vi "gcode_v2.vi"() -> ()   [LabVIEW 2020]
uses:
  bee2abb7-c490-4ad6-bfc0-30ed72578e14.vi
panel:
  in  "Convert":bool
  in  "Load":bool
  in  "File Path":path
  in  "Gcode":string
  out "Paths":cluster{"x":dbl, "y":dbl}[](array[cluster])
  out "Preview":cluster{dbl[], dbl[]}[](graph)
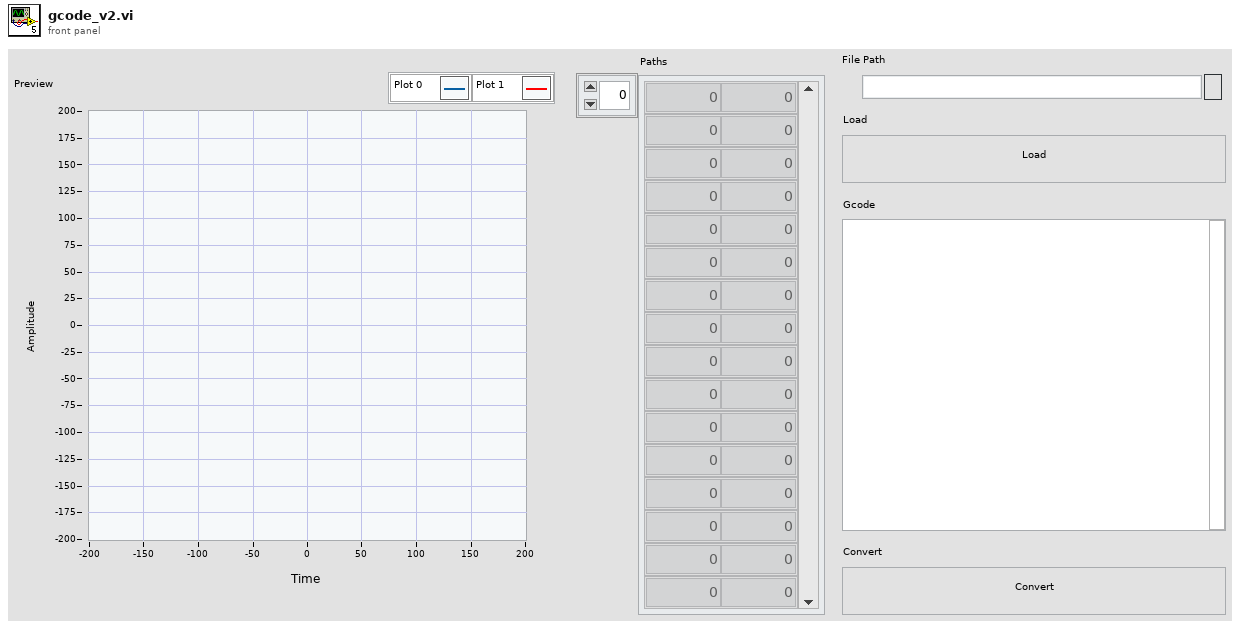
[diagram p1: front panel]
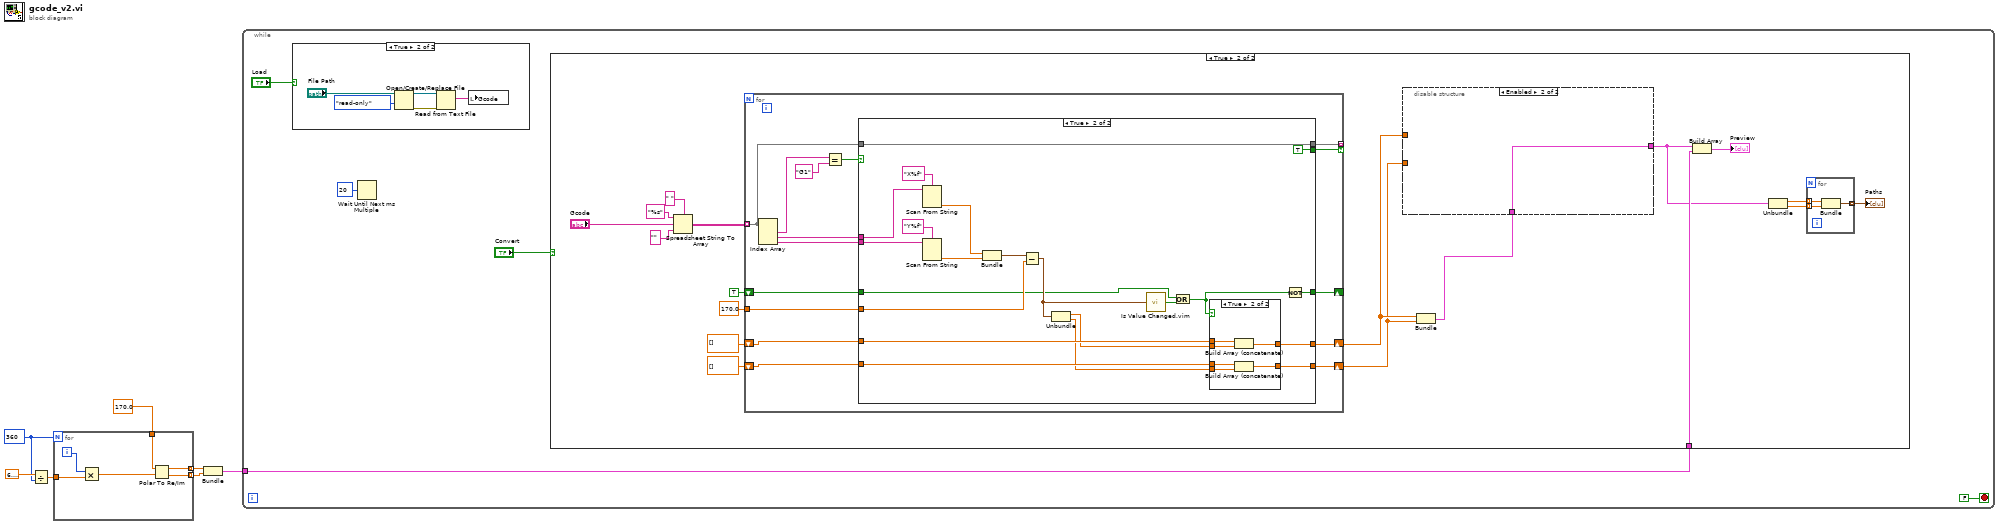
[diagram p0: block diagram]
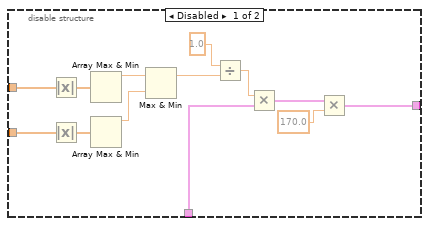
[diagram p5: hidden frame]
diagram:
  w6 = 360
  n1 = Divide(x=6.283185307179586, y=w6) -> (x/y=w5:dbl)
  n2 = for {
    N: w6 -> [_]
    tunnel: [w13] -> w3 mode=indexing
    tunnel: [w12] -> w2 mode=indexing
    tunnel: w5 -> [w10]
    tunnel: 170.0 ("r") -> [w8]
    i -> [w11]
    n3 = Multiply(x=w11, y=w10) -> (x*y=w9:dbl)
    n4 = Polar To Re/Im(2:w9, 3:w8) -> (0:w12:dbl, 1:w13:dbl)
  }
  n5 = Bundle(w3, w2) -> (w1:cluster{dbl[], dbl[]})  [unwired: 1 in]
  n6 = while {
    tunnel: w1 -> [w17]
    stop <- FALSE stop-if-true
    n7 = case shown="True" "Load" {
      frame False {
      }
      frame True {
        n8 = Open/Create/Replace File(file path (use dialog)="File Path", access (0:read/write)=enum16{"read/write", "read-only", "write-only"}."read-only") -> (refnum out=w102:refnum<file>, error out=w103:errorcluster)  [unwired: 4 in, 1 out]
        n9 = Read from Text File(file (use dialog)=w102, error in=w103) -> (text=w101:string)  [unwired: 2 in, 3 out]
        n10 = local write "Gcode"(w101) -> ()
      }
    }
    n11 = Wait Until Next ms Multiple(millisecond multiple=u32 20) -> ()  [unwired: 1 out]
    n12 = case shown="True" "Convert" {
      tunnel: w17 -> [_ w21]
      frame False {
      }
      frame True {
        n13 = Spreadsheet String To Array(delimiter (Tab)=" ", format string="%s", spreadsheet string="Gcode", array type (2D Dbl)="" ("delimiter (Tab)")) -> (array=w28:string[][])
        n14 = for {
          shift-right: [w49] -> w26
          shift-left: dbl[] [] -> [w51]
          shift-right: [w48] -> w25
          shift-left: dbl[] [] -> [w50]
          tunnel: w28 -> [w40] mode=indexing
          tunnel: 170.0 -> [w45]
          tunnel: [w41] -> _ mode=indexing if=w39
          shift-right: [w38] -> _
          shift-left: TRUE -> [w37]
          n15 = Index Array(array=w40) -> (element #1=w44:string, element #2=w47:string, element #3=w46:string)  [unwired: 3 in]
          n16 = Equal?(x=w44, y="G1") -> (x = y?=w42:bool)
          n17 = case shown="True" w42 {
            tunnel: w51 -> [w54 w75]
            tunnel: w50 -> [w53 w74]
            tunnel: [w54 w73] -> w49
            tunnel: [w53 w72] -> w48
            tunnel: w47 -> [_ w68]
            tunnel: w46 -> [_ w67]
            tunnel: w45 -> [_ w64]
            tunnel: [_ w60] -> w41
            tunnel: w40 -> [_ w60]
            tunnel: [_ TRUE] -> w39
            tunnel: [w52 w55] -> w38
            tunnel: w37 -> [w52 w57]
            frame False {
            }
            frame True {
              n18 = Scan From String(format string="X%f", input string=w68) -> (output 1=w70:dbl)  [unwired: 3 in, 3 out]
              n19 = Scan From String(format string="Y%f", input string=w67) -> (output 1=w66:dbl)  [unwired: 3 in, 3 out]
              n20 = Bundle(w70, w66) -> (w65:cluster{dbl, dbl})  [unwired: 1 in]
              n21 = Subtract(x=w65, y=w64) -> (x-y=w63:cluster{dbl, dbl})
              n22 = Unbundle(w63) -> (w62:dbl, w61:dbl)
              n23 = call "Is Value Changed.vim"("value"=w63) -> ("changed or first call?"=w58:bool)
              n24 = Or(x=w57, y=w58) -> (x .or. y?=w56:bool)
              n25 = case shown="True" w56 {
                tunnel: w62 -> [_ w83]
                tunnel: w61 -> [_ w82]
                tunnel: [w77 w81] -> w73
                tunnel: [w76 w80] -> w72
                tunnel: w75 -> [w77 w79]
                tunnel: w74 -> [w76 w78]
                frame False {
                }
                frame True {
                  n26 = Build Array (concatenate)(w79, w83) -> (w81:dbl[])
                  n27 = Build Array (concatenate)(w78, w82) -> (w80:dbl[])
                }
              }
              n28 = Not(x=w56) -> (.not. x?=w55:bool)
            }
          }
        }
        n29 = Bundle(w26, w25) -> (w22:cluster{dbl[], dbl[]})  [unwired: 1 in]
        n30 = disable-structure shown="Enabled" {
          disable-tunnel: w26 -> [w96 _]
          disable-tunnel: w25 -> [w95 _]
          disable-tunnel: w22 -> [w87 w97]
          disable-tunnel: [w84 w97] -> w19
          frame Disabled {
            n31 = Absolute Value(x=w96) -> (abs(x)=w94:dbl[])
            n32 = Absolute Value(x=w95) -> (abs(x)=w93:dbl[])
            n33 = Array Max & Min(array=w94) -> (max value=w92:dbl)  [unwired: 3 out]
            n34 = Array Max & Min(array=w93) -> (max value=w91:dbl)  [unwired: 3 out]
            n35 = Max & Min(x=w92, y=w91) -> (max(x,y)=w90:dbl)  [unwired: 1 out]
            n36 = Divide(x=1.0, y=w90) -> (x/y=w88:dbl)
            n37 = Multiply(x=w88, y=w87) -> (x*y=w86:cluster{dbl[], dbl[]})
            n38 = Multiply(x=w86, y=170.0 ("x")) -> (x*y=w84:cluster{dbl[], dbl[]})
          }
          frame Enabled {
          }
        }
        n39 = Build Array(w19, w21) -> (→"Preview":cluster{dbl[], dbl[]}[])
        n40 = Unbundle(w19) -> (w34:dbl[], w33:dbl[])
        n41 = for {
          tunnel: w34 -> [w100] mode=indexing
          tunnel: w33 -> [w99] mode=indexing
          tunnel: [w98] -> w24 mode=indexing
          n42 = Bundle("x"=w100, "y"=w99) -> (w98:cluster{"x":dbl, "y":dbl})  [unwired: 1 in]
        }
        "Paths" <- w24
      }
    }
  }
